vi "Tote_Pos_Arb.vi"(0 "Ben":bool, 1 "Exit_Floor":bool, 2 "Exit":bool, 3 "Step":bool, 4 "Station":bool, 5 "Station_Station":bool, 6 "Store":bool, 7 "Store_Floor":bool, 8 "Pickup_2":bool, 9 "Pickup_2_Station":bool, 10 "Exit_Score":bool, 11 "Step_Step":bool, 12 "Carry":bool, 13 "Step_3":bool, 16 "Step_1":bool, 18 "Store High":bool) -> (14 "Pos_Active":bool, 15 "Pos_Des":dbl)   [LabVIEW 2014]
panel:
  in  "Store_High_Val":dbl=35.0 format="%#_13g"
  in  "Step_1_Val":dbl=28.0 format="%#_13g"
  in  "Step_3_Val":dbl=53.0 format="%#_13g"
  in  "Carry_Val":dbl=12.5 format="%#_13g"
  in  "Pickup_2_Val":dbl=21.0 format="%#_13g"
  in  "Store_Val":dbl=24.0 format="%#_13g"
  in  "Tote_Feeder_Val":dbl=45.0 format="%#_13g"
  in  "Step_Val":dbl=18.0 format="%#_13g"
  in  "Exit_Val":dbl=8.25 format="%#_13g"
  in  "Ben_Val":dbl=8.0 format="%#_13g"
  # "1Ft 8in wide X 2 in Tall X 15 ft 7 in long"
  # "72 in"
  # "6"
  # "60 in"
  # "5"
  # "54.25 in"
  # "48 in"
  # "4"
  # "4"
  # "42.25 in"
  # "26.9in long X 16.9 in wide X 12.1 in Tall"
  # "36 in"
  # "3"
  # "3"
  # "30.25 in"
  # "2"
  # "24 in"
  # "1ft 6 in"
  # "18.25 in"
  # "2"
  # "1"
  # "12 in"
  # "1"
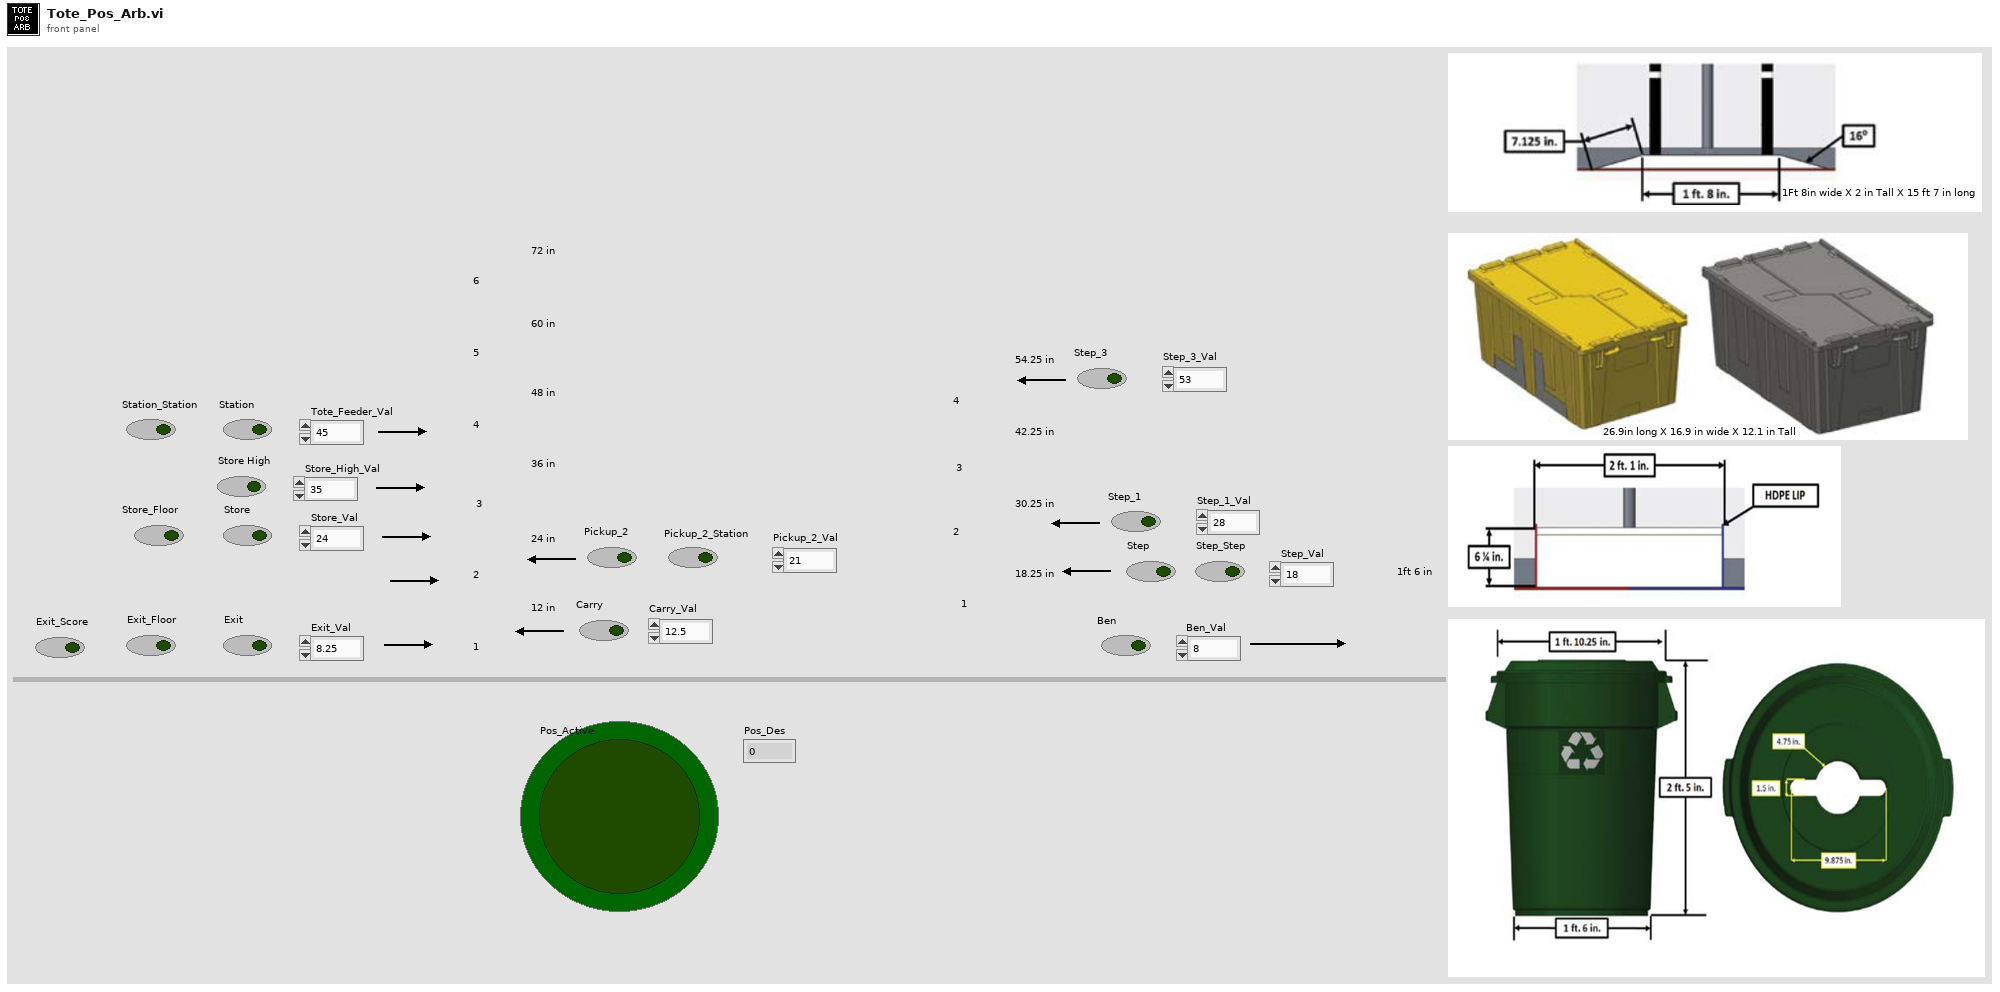
[diagram p1: front panel]
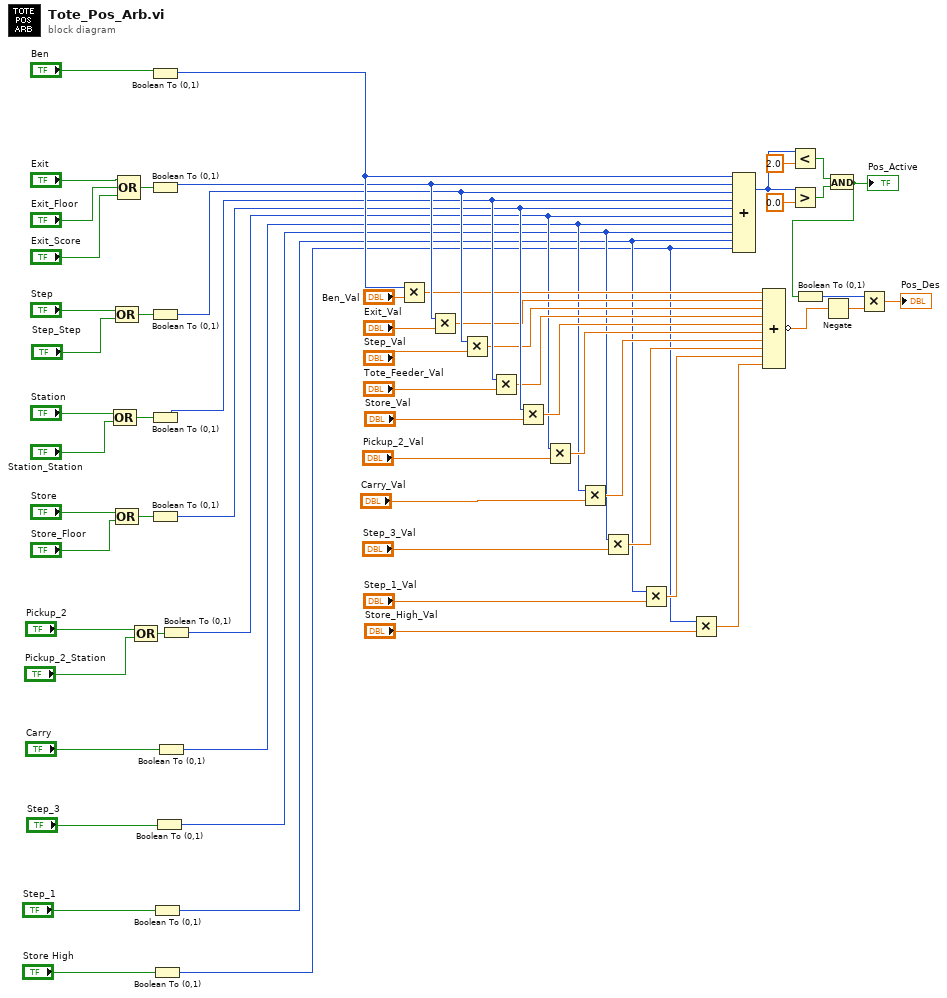
[diagram p0: block diagram]
diagram:
  n1 = Compound Arithmetic op=OR("Station", "Station_Station") -> (w28:bool)
  n2 = Compound Arithmetic op=OR("Step", "Step_Step") -> (w20:bool)
  n3 = Compound Arithmetic op=OR("Store", "Store_Floor") -> (w36:bool)
  n4 = Compound Arithmetic op=OR("Exit", "Exit_Floor", "Exit_Score") -> (w33:bool)
  n5 = Compound Arithmetic op=OR("Pickup_2", "Pickup_2_Station") -> (w25:bool)
  n6 = Boolean To (0,1)(Boolean="Ben") -> (0, 1=w55:i16)
  n7 = Boolean To (0,1)(Boolean=w33) -> (0, 1=w54:i16)
  n8 = Boolean To (0,1)(Boolean=w20) -> (0, 1=w53:i16)
  n9 = Boolean To (0,1)(Boolean=w28) -> (0, 1=w52:i16)
  n10 = Boolean To (0,1)(Boolean=w36) -> (0, 1=w51:i16)
  n11 = Boolean To (0,1)(Boolean="Step_1") -> (0, 1=w7:i16)
  n12 = Boolean To (0,1)(Boolean="Store High") -> (0, 1=w3:i16)
  n13 = Boolean To (0,1)(Boolean="Step_3") -> (0, 1=w11:i16)
  n14 = Boolean To (0,1)(Boolean="Carry") -> (0, 1=w15:i16)
  n15 = Boolean To (0,1)(Boolean=w25) -> (0, 1=w23:i16)
  n16 = Multiply(x=w55, y="Ben_Val") -> (x*y=w50:dbl)
  n17 = Multiply(x=w54, y="Exit_Val") -> (x*y=w49:dbl)
  n18 = Multiply(x=w53, y="Step_Val") -> (x*y=w48:dbl)
  n19 = Multiply(x=w52, y="Tote_Feeder_Val") -> (x*y=w47:dbl)
  n20 = Multiply(x=w51, y="Store_Val") -> (x*y=w46:dbl)
  n21 = Multiply(x=w23, y="Pickup_2_Val") -> (x*y=w22:dbl)
  n22 = Multiply(x=w15, y="Carry_Val") -> (x*y=w14:dbl)
  n23 = Multiply(x=w11, y="Step_3_Val") -> (x*y=w10:dbl)
  n24 = Multiply(x=w7, y="Step_1_Val") -> (x*y=w6:dbl)
  n25 = Multiply(x=w3, y="Store_High_Val") -> (x*y=w1:dbl)
  n26 = Compound Arithmetic op=ADD(w55, w54, w53, w52, w51, w23, w15, w11, w7, w3) -> (w40:i16)
  n27 = Compound Arithmetic op=ADD(w50, w49, w48, w47, w46, w22, w14, w10, w6, w1) -> (invert w38:dbl)
  n28 = Less?(x=w40, y=2.0) -> (x < y?=w41:bool)
  n29 = Greater?(x=w40, y=0.0) -> (0:w43:bool)
  n30 = Negate(x=w38) -> (-x=w37:dbl)
  n31 = And(x=w41, y=w43) -> (x .and. y?=w39:bool)
  "Pos_Active" <- w39
  n32 = Boolean To (0,1)(Boolean=w39) -> (0, 1=w45:i16)
  n33 = Multiply(x=w45, y=w37) -> (x*y=→"Pos_Des":dbl)
